vi "AIT 664 - Read XML Attribute.vi"(0 "Attributes In":refnum<k20>, 5 "Attribute Name":string, 11 "error in (no error)":errorcluster) -> (4 "Attributes Out":refnum<k20>, 6 "Attribute Text":string, 15 "error out":errorcluster)   [LabVIEW 2013, in "AIT 664 Custom Device.lvlib"]
doc: "Given an attributes for an xml node and the attribute name extrax the attribute text."
uses:
  AIT 664 Custom Device.lvlib
  <vilib>/xml/Close Reference(Node).vi
  <resource>/objmgr/DOMUserDefRef.rc
  <vilib>/xml/NI_XML.lvlib
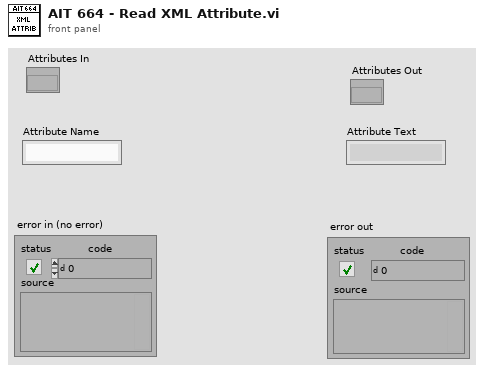
[diagram p1: front panel]
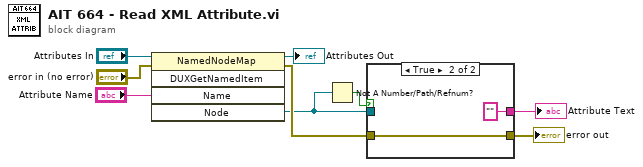
[diagram p0: block diagram]
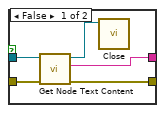
[diagram p2: hidden frame]
diagram:
  n1 = invoke on="Invoke Node" class="NamedNodeMap" method="DUXGetNamedItem"(reference="Attributes In", error in="error in (no error)", "Name"="Attribute Name") -> (reference out=→"Attributes Out":refnum<k20>, error out=w5:errorcluster, "Node"=w2:refnum<k20>)  [unwired: 2 in, 2 out]
  n2 = Not A Number/Path/Refnum?(number/path/refnum=w2) -> (NaN/Path/Refnum?=w1:bool)
  n3 = case shown="True" w1 {
    tunnel: [w14 "" ("node text")] -> w9
    tunnel: w2 -> [w13 _]
    tunnel: w5 -> [w12 w15]
    tunnel: [w11 w15] -> w4
    frame False {
      n4 = call <vilib>:"Get Node Text Content.vi"("error in (no error)"=w12, "node in"=w13) -> ("error out"=w11:errorcluster, "node text"=w14:string, "node out"=w10:refnum<k20>)  [unwired: 7 in]
      n5 = call-poly <vilib>:"Close.vi"("node"=w10) -> ()  [unwired: 8 in, 1 out]
    }
    frame True {
    }
  }
  "Attribute Text" <- w9
  "error out" <- w4
